vi "config_Burst.vi"(8 "error in (no error)":errorcluster, 9 "# ciclos":i32, 10 "Amplitud (Vrms)":dbl, 11 "Frec (Hz)":dbl) -> (0 "error out":errorcluster, 3 "DS360 out":refnum<class "DS360.lvclass">)   [LabVIEW 2019, in "DS360.lvclass"]
uses:
  DS360.lvclass
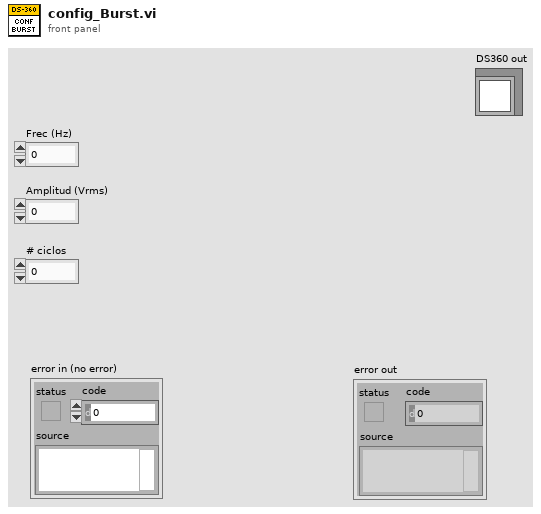
[diagram p1: front panel]
types:
  T1 = cluster{"error":bool, "code":i32, "source":string}
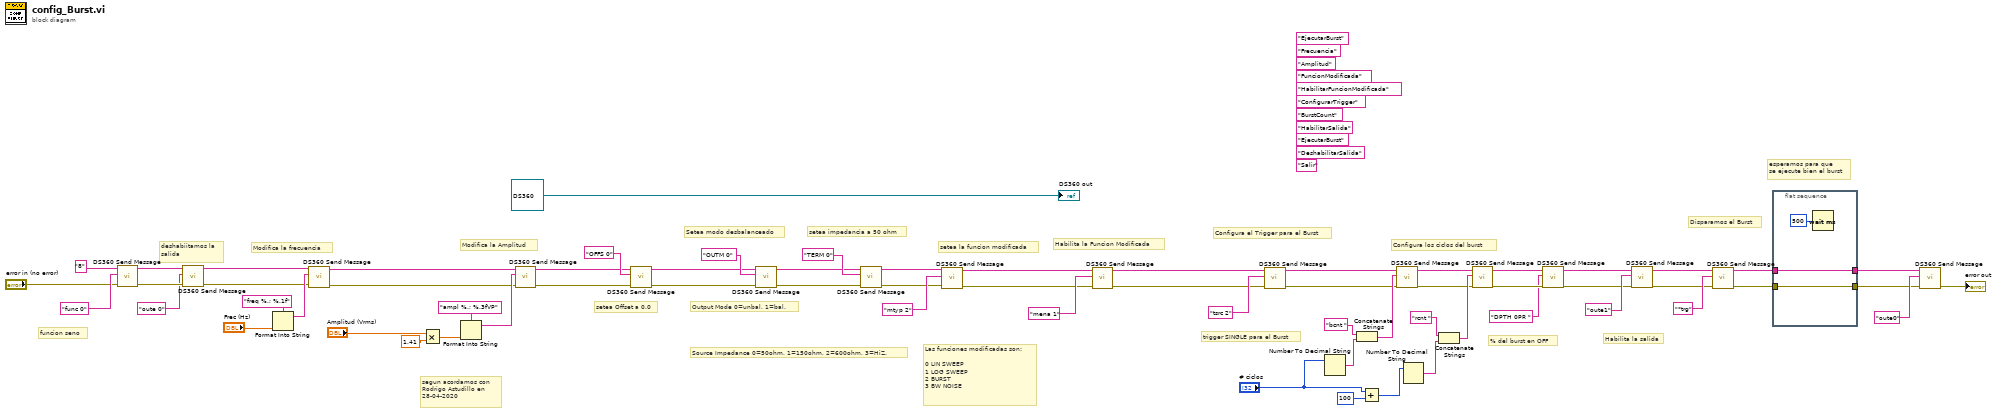
[diagram p0: block diagram]
diagram:
  (unwired) "Salir"
  (unwired) "DeshabilitarSalida"
  (unwired) "EjecutarBurst"
  (unwired) "HabilitarSalida"
  (unwired) "BurstCount"
  (unwired) "ConfigurarTrigger"
  (unwired) "HabilitarFuncionModificada"
  (unwired) "FuncionModificada"
  (unwired) "Amplitud"
  (unwired) "Frecuencia"
  (unwired) "EjecutarBurst"
  # "deshabiitamos la \nsalida"
  # "Source Impedance 0=50ohm, 1=150ohm, 2=600ohm, 3=HiZ."
  # "Output Mode 0=unbal, 1=bal."
  # "setea impedancia a 50 ohm"
  # "Setea modo desbalanceado"
  # "setea Offset a 0.0"
  # "% del burst en OFF"
  # "Las funciones modificadas son:\n\n0 LIN SWEEP\n1 LOG SWEEP\n2 BURST\n3 BW NOISE"
  # "funcion seno"
  # "esperamos para que\nse ejecute bien el burst"
  # "Disparamos el Burst"
  # "Habilita la salida"
  # "Configura los ciclos del burst"
  # "trigger SINGLE para el Burst"
  # "Configura el Trigger para el Burst"
  # "Habilita la Funcion Modificada"
  # "setea la funcion modificada"
  # "Modifica la Amplitud"
  # "segun acordamos con\nRodrigo Astudillo en\n28-04-2020"
  # "Modifica la frecuencia"
  n1 = call <instrlib>:"DS360 Send Message.vi"("address string"="8" ("write buffer"), "write buffer"="func 0", "error in"="error in (no error)") -> ("address out"=w5:string, "error out"=w3:T1)  [unwired: 3 in, 2 out]
  n2 = call <instrlib>:"DS360 Send Message.vi"("address string"=w5, "write buffer"="oute 0", "error in"=w3) -> ("address out"=w4:string, "error out"=w2:T1)  [unwired: 3 in, 2 out]
  n3 = Format Into String(format string="freq %.; %.1f" ("write buffer"), "Frec (Hz)") -> (resulting string=w61:string)  [unwired: 2 in, 1 out]
  n4 = call <instrlib>:"DS360 Send Message.vi"("address string"=w4, "write buffer"=w61, "error in"=w2) -> ("address out"=w36:string, "error out"=w37:T1)  [unwired: 3 in, 2 out]
  n5 = Multiply(x="Amplitud (Vrms)", y=1.41) -> (x*y=w58:dbl)
  n6 = Format Into String(format string="ampl %.; %.3fVP" ("write buffer"), w58) -> (resulting string=w56:string)  [unwired: 2 in, 1 out]
  n7 = call <instrlib>:"DS360 Send Message.vi"("address string"=w36, "write buffer"=w56, "error in"=w37) -> ("address out"=w11:string, "error out"=w10:T1)  [unwired: 3 in, 2 out]
  n8 = call <instrlib>:"DS360 Send Message.vi"("address string"=w11, "write buffer"="OFFS 0", "error in"=w10) -> ("address out"=w7:string, "error out"=w15:T1)  [unwired: 3 in, 2 out]
  n9 = call <instrlib>:"DS360 Send Message.vi"("address string"=w7, "write buffer"="OUTM 0", "error in"=w15) -> ("address out"=w6:string, "error out"=w14:T1)  [unwired: 3 in, 2 out]
  n10 = call <instrlib>:"DS360 Send Message.vi"("address string"=w6, "write buffer"="TERM 0", "error in"=w14) -> ("address out"=w9:string, "error out"=w8:T1)  [unwired: 3 in, 2 out]
  n11 = call <instrlib>:"DS360 Send Message.vi"("address string"=w9, "write buffer"="mtyp 2", "error in"=w8) -> ("address out"=w34:string, "error out"=w33:T1)  [unwired: 3 in, 2 out]
  n12 = call <instrlib>:"DS360 Send Message.vi"("address string"=w34, "write buffer"="mena 1", "error in"=w33) -> ("address out"=w32:string, "error out"=w31:T1)  [unwired: 3 in, 2 out]
  n13 = call <instrlib>:"DS360 Send Message.vi"("address string"=w32, "write buffer"="tsrc 2", "error in"=w31) -> ("address out"=w30:string, "error out"=w29:T1)  [unwired: 3 in, 2 out]
  n14 = Number To Decimal String(number="# ciclos") -> (decimal integer string=w43:string)  [unwired: 1 in]
  n15 = Concatenate Strings("bcnt " ("write buffer"), w43) -> (w51:string)
  n16 = Add(x="# ciclos", y=100) -> (x+y=w47:i32)
  n17 = call <instrlib>:"DS360 Send Message.vi"("address string"=w30, "write buffer"=w51, "error in"=w29) -> ("address out"=w44:string, "error out"=w45:T1)  [unwired: 3 in, 2 out]
  n18 = Number To Decimal String(number=w47) -> (decimal integer string=w50:string)  [unwired: 1 in]
  n19 = Concatenate Strings("rcnt " ("write buffer"), w50) -> (w49:string)
  n20 = call <instrlib>:"DS360 Send Message.vi"("address string"=w44, "write buffer"=w49, "error in"=w45) -> ("address out"=w21:string, "error out"=w20:T1)  [unwired: 3 in, 2 out]
  n21 = call <instrlib>:"DS360 Send Message.vi"("address string"=w21, "write buffer"="DPTH 0PR ", "error in"=w20) -> ("address out"=w17:string, "error out"=w18:T1)  [unwired: 3 in, 2 out]
  n22 = call <instrlib>:"DS360 Send Message.vi"("address string"=w17, "write buffer"="oute1", "error in"=w18) -> ("address out"=w28:string, "error out"=w27:T1)  [unwired: 3 in, 2 out]
  n23 = call <instrlib>:"DS360 Send Message.vi"("address string"=w28, "write buffer"="*trg", "error in"=w27) -> ("address out"=w26:string, "error out"=w25:T1)  [unwired: 3 in, 2 out]
  n24 = flat-sequence {
    tunnel: w26 -> [w67]
    tunnel: w25 -> [w66]
    tunnel: [w67] -> w24
    tunnel: [w66] -> w23
    frame #0 {
      n25 = Wait (ms)(milliseconds to wait=u32 500) -> ()  [unwired: 1 out]
    }
  }
  n26 = call <instrlib>:"DS360 Send Message.vi"("address string"=w24, "write buffer"="oute0", "error in"=w23) -> ("error out"=→"error out":T1)  [unwired: 3 in, 3 out]
  "DS360 out" <- refnum<class "DS360.lvclass"> refnum ("DS360 in")
